vi "CC Observation to Script.vi"(8 "error in (no error)":errorcluster, 11 "Observation":T3={"Priority"=0, "ID"="", "Observer"="", "Obj Name"="", "Obj Type"="", "RA and DEC String"={"RA"="HH:MM:SS.nnn", "DEC"="DEG:arcmin:arcsec.nn"}, "Filter Wheel 1"="", "Filter Wheel 2"="", "Integration Time"=0.0, "Observation Status"=enum."Error", "Offsets"={"RA"=0.0, "DEC"=0.0, "ROT"=0.0}, "Images"=0, "Dither Options"={"Dither"=enum."None", "Dither Radius"=0.0, "Dither Points"=0, "Dither Phase"=0.0}, "Comment 1"="", "Comment 2"=""}) -> (0 "error out":errorcluster, 3 "Script Steps":T1[](array[typedef]))   [LabVIEW 2021]
uses:
  typedefs/CC cluster Observation.ctl
  Observation Queue/CC enum Observation Status.ctl
  Telescope/CC cluster Telescope Offsets.ctl
  typedefs/CC cluster Observation Dither Options.ctl
  typedefs/CC enum Dither Selection.ctl
  typedefs/CC Script Step.ctl
  typedefs/CC enum Script Action.ctl
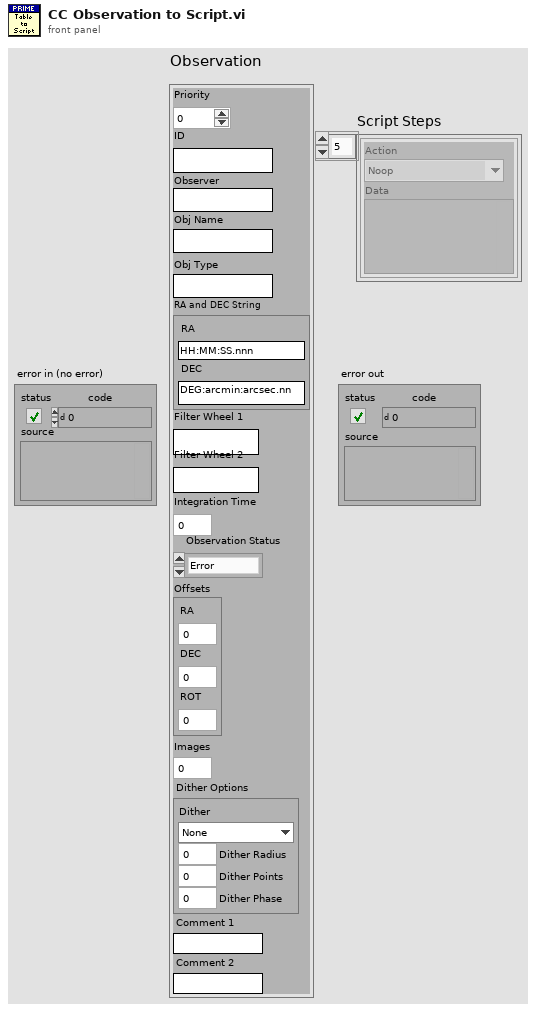
[diagram p1: front panel]
types:
  T1 = typedef "CC Script Step.ctl" = cluster{"Action":T2, "Data":variant}
  T2 = typedef "CC enum Script Action.ctl" = enum16{"Noop", "Define Object", "Define Exposure", "Define Dithering", "Acquire Images", "Set Filter Wheel", "Telescope Home", "Telescope Move", "Telescope RA DEC", "Focus Move Relative", "Focus Move Absolute", "Focus Set Home", "Macro", "Pause", "Ask User", "Define Random Dither"}
  T3 = typedef "CC cluster Observation.ctl" = cluster{"Priority":i32, "ID":string, "Observer":string, "Obj Name":string, "Obj Type":string, "RA and DEC String":cluster{"RA":string, "DEC":string}, "Filter Wheel 1":string, "Filter Wheel 2":string, "Integration Time":dbl, "Observation Status":T4, "Offsets":T5, "Images":i32, "Dither Options":T6, "Comment 1":string, "Comment 2":string}
  T4 = typedef "CC enum Observation Status.ctl" = enum16{"Ready", "Running", "Done", "Error"}
  T5 = typedef "CC cluster Telescope Offsets.ctl" = cluster{"RA":dbl, "DEC":dbl, "ROT":dbl}
  T6 = typedef "CC cluster Observation Dither Options.ctl" = cluster{"Dither":T7, "Dither Radius":dbl, "Dither Points":i32, "Dither Phase":dbl}
  T7 = typedef "CC enum Dither Selection.ctl" = enum16{"None", "Circle", "Random"}
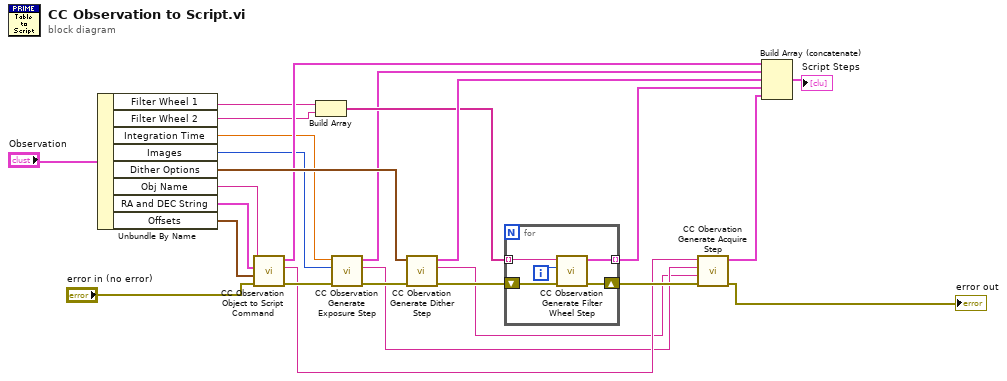
[diagram p0: block diagram]
diagram:
  n1 = Unbundle By Name("Observation") -> ("Filter Wheel 1"=w20:string, "Filter Wheel 2"=w19:string, "Integration Time"=w16:dbl, "Images"=w1:i32, "Dither Options"=w22:T6, "Obj Name"=w12:string, "RA and DEC String"=w13:cluster{"RA":string, "DEC":string}, "Offsets"=w14:T5)
  n2 = call "CC Observation Object to Script Command.vi"("error in (no error)"="error in (no error)", "Offsets"=w14, "RA and DEC String"=w13, "Object.Name"=w12) -> ("error out"=w11:errorcluster, "Object Name out"=w4:string, "Define Object Step"=w21:T1)  [unwired: 5 in]
  n3 = Build Array(w20, w19) -> (w18:string[])
  n4 = call "CC Observation Generate Exposure Step.vi"("error in (no error)"=w11, "Images"=w1, "Integration Time"=w16) -> ("error out"=w10:errorcluster, "Exp Name"=w3:string, "Exp Step"=w15:T1)  [unwired: 6 in]
  n5 = call "CC Obervation Generate Dither Step.vi"("error in (no error)"=w10, "Dither Options"=w22) -> ("error out"=w9:errorcluster, "Name"=w2:string, "Step"=w23:T1)  [unwired: 7 in]
  n6 = for {
    tunnel: w18 -> [w30] mode=indexing
    tunnel: [w28] -> w17 mode=indexing
    shift-right: [w26] -> w7
    shift-left: w9 -> [w27]
    i -> [w29]
    n7 = call "CC Observation Generate Filter Wheel Step.vi"("error in (no error)"=w27, "Wheel (0 or 1)"=w29, "Filter Wheel Name"=w30) -> ("error out"=w26:errorcluster, "Step"=w28:T1)  [unwired: 7 in]
  }
  n8 = call "CC Obervation Generate Acquire Step.vi"("error in (no error)"=w7, "Dithering"=w2, "Exposure"=w3, "Object"=w4) -> ("error out"=→"error out":errorcluster, "Acquire Step"=w5:T1)  [unwired: 6 in]
  n9 = Build Array (concatenate)(w21, w15, w23, w17, w5) -> (→"Script Steps":T1[])
